vi "minJerk.vi"(8 "tf":dbl, 9 "t":dbl, 10 "Xf":dbl, 11 "Xi":dbl) -> (2 "Xnext":dbl)   [LabVIEW 2018]
uses:
  <vilib>/imath/engines/lvmath2/RunTimeEngine/NodeEndStatement/NIMS_NodeEndStatement_Output.vi
  <instcachedir>/0/NIMS_NodeEndStatement_Output_53EC0D466D134D7ABD903AC30B43404B.lvgen/NIMS_NodeEndStatement_Output_53EC0D466D134D7ABD903AC30B43404B_001.vi
  <vilib>/imath/engines/lvmath2/RunTimeEngine/ErrorHandling/NIMS_Finalize Error.vi
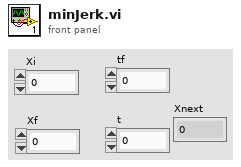
[diagram p1: front panel]
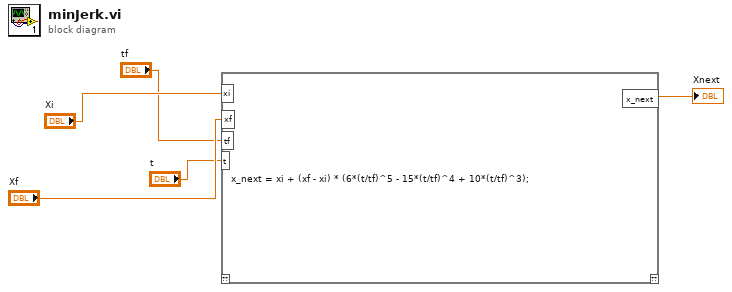
[diagram p0: block diagram]
diagram:
  n1 = mathscript code="x_next = xi + (xf - xi) * (6*(t/tf)^5 - 15*(t/tf)^4 + 10*(t/tf)^3);"("xi"="Xi", "xf"="Xf", "tf"="tf", "t"="t") -> ("x_next"=→"Xnext":dbl)  [unwired: 1 in, 1 out]
